vi "Memory.Pointer.Dispose.vi"(8 "error in (no error)":errorcluster, 11 "Pointer in":refnum<class "Memory.Pointer.Void.lvclass">) -> (0 "error out":errorcluster)   [LabVIEW 2016, in "Memory.Pointer.Void.lvclass"]
uses:
  Memory.Pointer.Void.lvclass
  Memory.Pointer.Void.lvclass/Memory.Pointer.Void.ctl
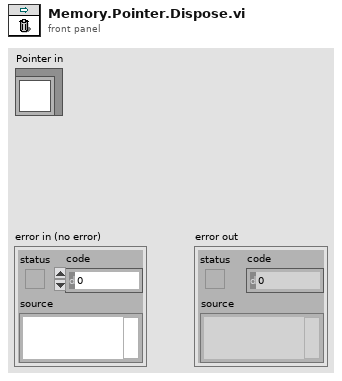
[diagram p1: front panel]
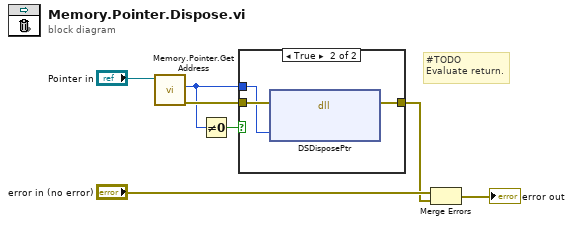
[diagram p0: block diagram]
diagram:
  # "#TODO\nEvaluate return."
  n1 = call "Memory.Pointer.Get Address.vi"("Pointer in"="Pointer in") -> ("error out"=w7:errorcluster, "address"=w6:u64)  [unwired: 8 in, 1 out]
  n2 = Not Equal To 0?(x=w6) -> (x != 0?=w5:bool)
  n3 = case shown="True" w5 {
    tunnel: w7 -> [w8 w11]
    tunnel: [w8 w10] -> w3
    tunnel: w6 -> [_ w9]
    frame False {
    }
    frame True {
      n4 = dll-call lib="LabVIEW" fn="DSDisposePtr"(error in=w11, "pointer"=w9) -> (error out=w10:errorcluster)  [unwired: 4 in, 1 out]
    }
  }
  n5 = Merge Errors("error in (no error)", w3) -> (→"error out":errorcluster)
